vi "OpenSlide.vi"(0 "Slide":string) -> ()   [LabVIEW 2014]
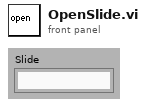
[diagram p1: front panel]
types:
  T1 = typedef "LVRectTypeDef.ctl" = cluster{"Left":i16, "Top":i16, "Right":i16, "Bottom":i16}
  T2 = cluster{"Left":i16, "Top":i16, "Left":i16, "Top":i16}
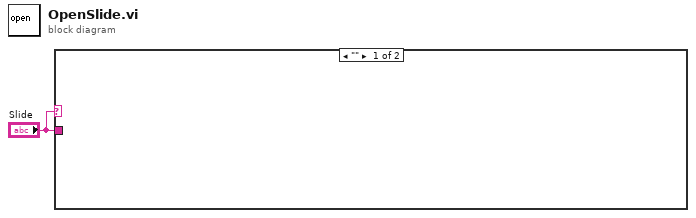
[diagram p0: block diagram]
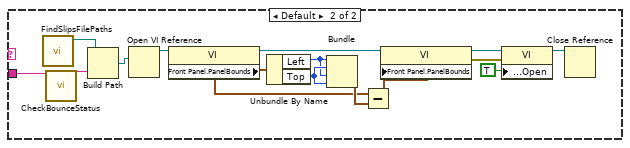
[diagram p2: hidden frame]
diagram:
  n1 = case shown="\"\"" "Slide" {
    tunnel: "Slide" -> [_ w3]
    frame "" {
    }
    frame Default {
      n2 = call "FindSlipsFilePaths.vi"() -> ("Slides"=w4:path)  [unwired: 2 in, 4 out]
      n3 = call "CheckBounceStatus.vi"("File Name"=w3) -> ("file name"=w2:string)  [unwired: 1 in, 2 out]
      n4 = Build Path(base path=w4, name or relative path=w2) -> (appended path=w5:path)
      n5 = Open VI Reference(vi path=w5) -> (vi reference=w8:refnum<vi>)  [unwired: 5 in, 1 out]
      n6 = property class="VI"(reference=w8) -> (reference out=w9:refnum<vi>, "Front Panel.PanelBounds"=w10:T1)  [unwired: 1 in, 1 out]
      n7 = Unbundle By Name(w10) -> ("Left"=w6:i16, "Top"=w7:i16)
      n8 = Bundle("Left"=w6, "Top"=w7, "Left"=w6, "Top"=w7) -> (w11:T2)  [unwired: 1 in]
      n9 = Subtract(x=w10, y=w11) -> (x-y=w12:T1)
      n10 = property class="VI"(reference=w9, "Front Panel.PanelBounds"=w12) -> (reference out=w13:refnum<vi>, error out=w14:errorcluster)  [unwired: 1 in]
      n11 = property class="VI"(reference=w13, error in=w14, "Front Panel.Open"=TRUE ("Front Panel Window:Open")) -> (reference out=w16:refnum<vi>)  [unwired: 1 out]
      n12 = Close Reference(reference=w16) -> ()  [unwired: 1 in, 1 out]
    }
  }
